vi "Close.vi"(8 "error in (no error)":errorcluster, 11 "Hioki BT4560B":refnum<class "Hioki BT4560B.lvclass">) -> (0 "error out":errorcluster, 3 "Hioki BT4560B out":refnum<class "Hioki BT4560B.lvclass">)   [LabVIEW 2025, in "ACIR.lvlib" / "Hioki BT4560B.lvclass"]
uses:
  Hioki BT4560B.lvclass
  Hioki BT4560B.lvclass/Hioki BT4560B.ctl
  <instrlib>/HIOKI BT4560/HIOKI BT4560.lvlib
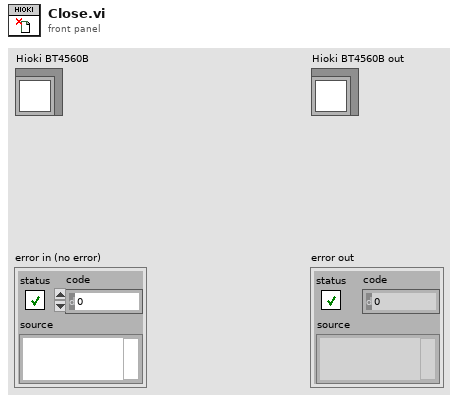
[diagram p1: front panel]
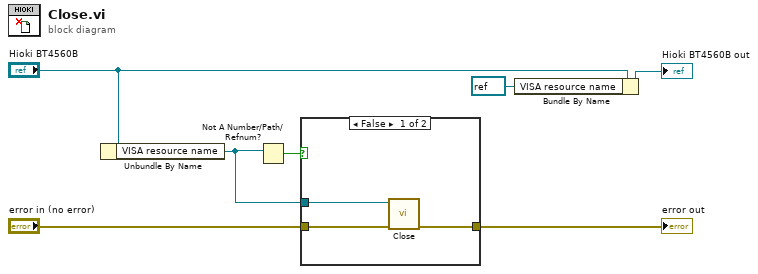
[diagram p0: block diagram]
diagram:
  n1 = Unbundle By Name("Hioki BT4560B") -> ("VISA resource name"=w6:refnum<visa-resource-name>)
  n2 = Not A Number/Path/Refnum?(number/path/refnum=w6) -> (NaN/Path/Refnum?=w7:bool)
  n3 = case shown="False" w7 {
    tunnel: [w9 w11] -> w2
    tunnel: "error in (no error)" -> [w10 w11]
    tunnel: w6 -> [w8 _]
    frame False {
      n4 = call <instrlib>:"Close.vi"("error in (no error)"=w10, "VISA resource name"=w8) -> ("error out"=w9:errorcluster)  [unwired: 9 in]
    }
    frame True {
    }
  }
  "error out" <- w2
  n5 = Bundle By Name(cluster="Hioki BT4560B", "VISA resource name"=refnum<visa-resource-name> refnum) -> (→"Hioki BT4560B out":refnum<class "Hioki BT4560B.lvclass">)
